vi "svc_Color Converter.vi"(11 "BG color":u32(colorbox)) -> (0 "low contrast":u32(colorbox), 1 "RGB compliment":u32(colorbox), 2 "maximum contrast":u32(colorbox), 3 "grayscale":u32(colorbox))   [LabVIEW 2017]
panel:
  in  "low contrast offset":u8=32 step=1
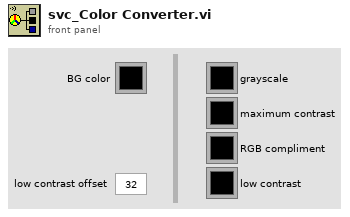
[diagram p1: front panel]
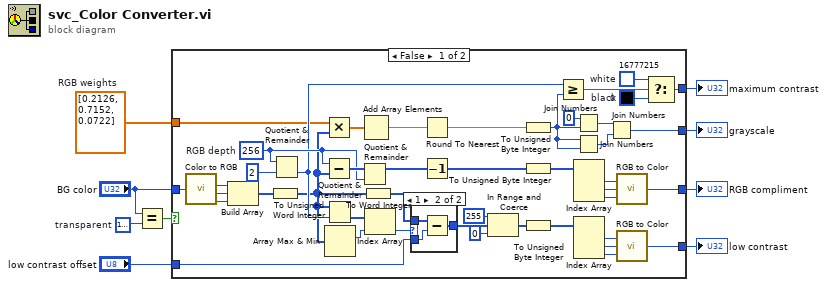
[diagram p0: block diagram]
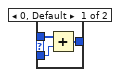
[diagram p2: hidden frame]
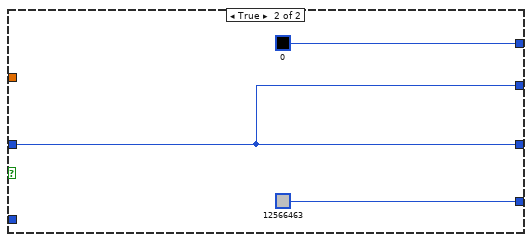
[diagram p3: hidden frame]
diagram:
  w1 = dbl[] [0.2126, 0.7152, 0.0722]  # RGB weights
  w7 = u32 16777216  # transparent
  n1 = Equal?(x="BG color", y=w7) -> (x = y?=w5:bool)
  n2 = case shown="False" w5 {
    tunnel: [w51 u32 12566463 ("maximum contrast")] -> w9
    tunnel: [w39 w60] -> w8
    tunnel: [w28 u32 0 ("maximum contrast")] -> w4
    tunnel: "BG color" -> [w38 w60]
    tunnel: [w22 w60] -> w3
    tunnel: "low contrast offset" -> [w16 _]
    tunnel: w1 -> [w10 _]
    frame False {
      w30 = u32 16777215  # white
      w29 = u32 0  # black
      w37 = u16 256  # RGB depth
      n3 = call <vilib>:"Color to RGB.vi"("Color"=w38) -> ("R"=w42:u8, "G"=w43:u8, "B"=w44:u8)  [unwired: 1 out]
      n4 = Build Array(w42, w43, w44) -> (w40:u8[])
      n5 = To Unsigned Word Integer(number=w40) -> (unsigned 16bit integer=w17:u16[])
      n6 = Quotient & Remainder(x=w37, y=u16 2) -> (floor(x/y)=w32:u16)  [unwired: 1 out]
      n7 = Multiply(x=w10, y=w17) -> (x*y=w34:dbl[])
      n8 = Subtract(x=w37, y=w17) -> (x-y=w41:u16[])
      n9 = Quotient & Remainder(x=w17, y=w32) -> (floor(x/y)=w20:u16[])  [unwired: 1 out]
      n10 = Array Max & Min(array=w17) -> (max index (indices)=w19:i32)  [unwired: 3 out]
      n11 = Quotient & Remainder(x=w41, y=w37) -> (x-y*floor(x/y)=w52:u16[])  [unwired: 1 out]
      n12 = Add Array Elements(numeric array=w34) -> (sum=w33:dbl)
      n13 = To Word Integer(number=w17) -> (16bit integer=w14:i16[])
      n14 = Index Array(array=w20, index=w19) -> (element=w18:u16)
      n15 = case shown="1" w18 {
        tunnel: w14 -> [w55 w59]
        tunnel: w16 -> [w54 w58]
        tunnel: [w56 w57] -> w15
        frame 0, Default {
          n16 = Add(x=w55, y=w54) -> (x+y=w56:i16[])
        }
        frame 1 {
          n17 = Subtract(x=w59, y=w58) -> (x-y=w57:i16[])
        }
      }
      n18 = Round To Nearest(number=w33) -> (nearest integer value=w26:dbl)
      n19 = Decrement(x=w52) -> (x-1=w27:u16[])
      n20 = In Range and Coerce(upper limit=i16 255 ("RGB depth"), x=w15, lower limit=i16 0 ("RGB depth")) -> (coerced(x)=w13:i16[])  [unwired: 1 out]
      n21 = To Unsigned Byte Integer(number=w26) -> (unsigned 8bit integer=w21:u8)
      n22 = To Unsigned Byte Integer(number=w27) -> (unsigned 8bit integer=w53:u8[])
      n23 = To Unsigned Byte Integer(number=w13) -> (unsigned 8bit integer=w35:u8[])
      n24 = Greater Or Equal?(x=w32, y=w21) -> (x >= y?=w31:bool)
      n25 = Join Numbers(hi=u8 0, lo=w21) -> ((hi.lo)=w25:u16)
      n26 = Join Numbers(hi=w21, lo=w21) -> ((hi.lo)=w24:u16)
      n27 = Index Array(array=w53) -> (element #1=w45:u8, element #2=w46:u8, element #3=w47:u8)  [unwired: 3 in]
      n28 = Index Array(array=w35) -> (element #1=w50:u8, element #2=w49:u8, element #3=w48:u8)  [unwired: 3 in]
      n29 = Join Numbers(hi=w25, lo=w24) -> ((hi.lo)=w22:u32)
      n30 = call <vilib>:"RGB to Color.vi"("B"=w47, "G"=w46, "R"=w45) -> ("Color"=w39:u32)
      n31 = call <vilib>:"RGB to Color.vi"("B"=w48, "G"=w49, "R"=w50) -> ("Color"=w51:u32)
      n32 = Select(t=w30, s=w31, f=w29) -> (s? t:f=w28:u32)
    }
    frame True {
    }
  }
  "RGB compliment" <- w8
  "low contrast" <- w9
  "maximum contrast" <- w4
  "grayscale" <- w3
